vi "Config.vi"(8 "error in (no error)":errorcluster, 10 "Setting":variant, 11 "NI DMM in":refnum<class "NI DMM.lvclass">) -> (0 "error out":errorcluster, 3 "NI DMM out":refnum<class "NI DMM.lvclass">)   [LabVIEW 2025, in "DMM.lvlib" / "NI DMM.lvclass"]
uses:
  NI DMM.lvclass
  C:/Users/Public/Documents/Sandia National Labs/TSS Plugin/CEF.lvlibp/Node/CEF_Node.lvclass
  C:/Working copy/tss/Plugin/Engines/DMM/DMM Instrument/DMM Instrument.lvclass
  C:/Users/Public/Documents/Sandia National Labs/TSS Plugin/Abstract Engine.lvlibp/Abstract Instrument/Abstract Instrument.lvclass
  DMM configuration/DMM configuration.lvclass
  <instrlib>/niDMM/nidmm.llb/niDMM Function.ctl
  NI DMM.lvclass/NI DMM.ctl
  DMM configuration/DMM configuration.lvclass/DMM configuration.ctl
  <instrlib>/niDMM/nidmm.llb/niDMM Current Source.ctl
  <instrlib>/niDMM/nidmm.llb/niDMM Resolution in Digits.ctl
  Users/Public/Documents/Sandia National Labs/TSS Plugin/Abstract Engine.lvlibp/Abstract Instrument/Channel.ctl
  DMM Channel/DMM Channel.lvclass
  Users/Public/Documents/Sandia National Labs/TSS Plugin/Abstract Engine.lvlibp/Channel configuration/Channel configuration.lvclass
  DMM configuration/Read DMM Setting.vi
  Users/Public/Documents/Sandia National Labs/TSS Plugin/CEF.lvlibp/Node/ReadChildren.vi
  Users/Public/Documents/Sandia National Labs/TSS Plugin/Abstract Engine.lvlibp/Channel configuration/Read Channel Setting.vi
  <instrlib>/niDMM/nidmm.llb/niDMM Configure Measurement Digits.vi
  Users/Public/Documents/Sandia National Labs/TSS Plugin/CEF.lvlibp/Node/CEF_Node.lvclass
  Users/Public/Documents/Sandia National Labs/TSS Plugin/CEF.lvlibp/serializable configuration/CEF_serializable configuration.lvclass
  Users/Public/Documents/Sandia National Labs/TSS Plugin/Abstract Engine.lvlibp/Abstract Instrument/Abstract Instrument.lvclass
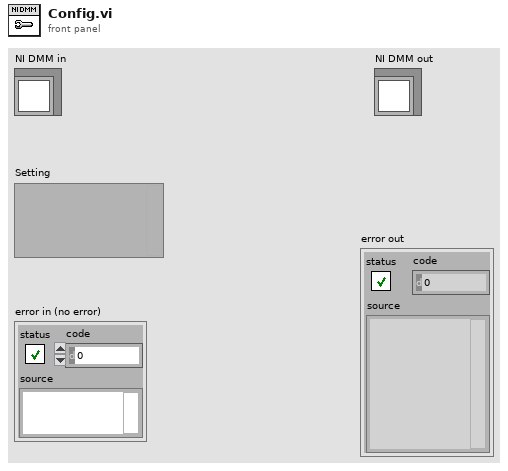
[diagram p1: front panel]
types:
  T1 = typedef "niDMM Function.ctl" = enum16{"DC Volts", "AC Volts", "DC Current", "AC Current", "2-wire Resistance", "4-wire Resistance", "Diode", "Frequency", "Period", "AC Volts DC Coupled", "Capacitance", "Inductance", "Temperature"}
  T2 = typedef "Abstract Engine.lvlibp/Abstract Instrument.lvclass/Channel.ctl" = cluster{"Alias":string, "DataType":enum16{"Anaolg Input", "Waveform"}, "Unit":enum16{"---", "V", "A", "Ohm", "Hz", "uF", "degC", "deg"}, "Upper limit":dbl, "Lower limit":dbl, "Measurement":variant}
  T3 = typedef "Abstract Engine.lvlibp/Channel configuration.lvclass/Default Channel.ctl" = cluster{"Address":string, "SW Alias":string, "Enabled":bool, "Type":string, "Description":string}
  T4 = typedef "DMM.lvlib/DMM configuration.lvclass/DMM Setting.ctl" = cluster{"Function":string, "CurrentSource":string, "Resolution":string, "Range":dbl}
  T5 = typedef "niDMM Resolution in Digits.ctl" = dbl
  T6 = typedef "niDMM Current Source.ctl" = dbl
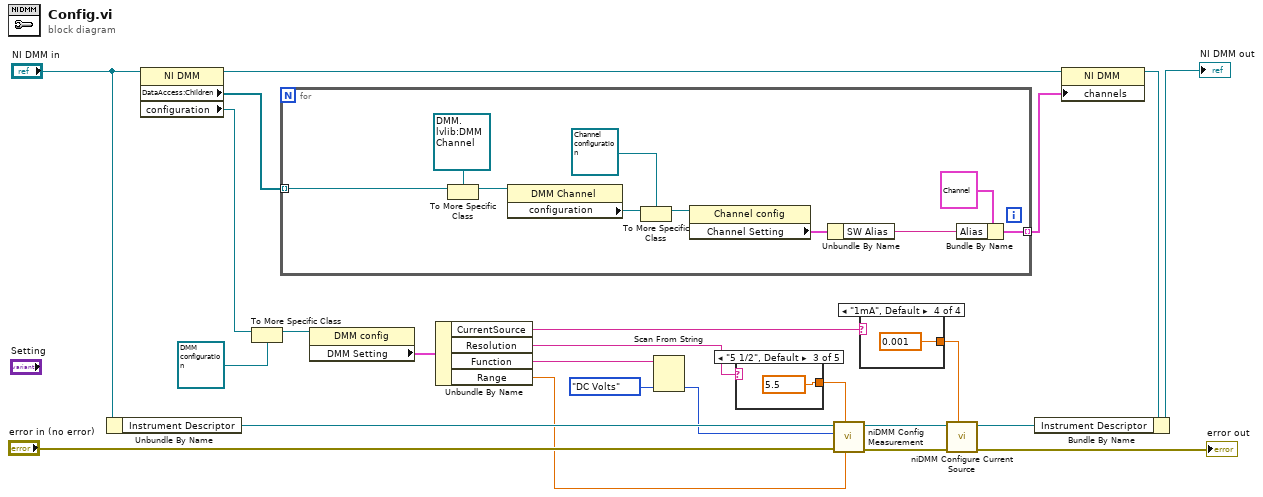
[diagram p0: block diagram]
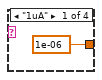
[diagram p2: hidden frame]
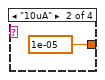
[diagram p3: hidden frame]
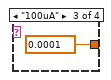
[diagram p4: hidden frame]
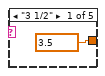
[diagram p5: hidden frame]
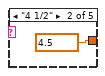
[diagram p6: hidden frame]
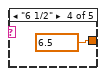
[diagram p7: hidden frame]
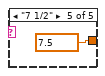
[diagram p8: hidden frame]
diagram:
  n1 = Unbundle By Name("NI DMM in") -> ("Instrument Descriptor"=w23:refnum<k15>)
  n2 = property class="NI DMM"(reference="NI DMM in") -> (reference out=w17:refnum<class "NI DMM.lvclass">, "DataAccess:Children"=w5:refnum<data-value>[], "configuration"=w6:refnum<class "CEF_serializable configuration.lvclass">)  [unwired: 1 in, 1 out]
  n3 = To More Specific Class(target class=refnum<class "DMM configuration.lvclass"> refnum ("DMM.lvlib:DMM configuration.lvclass"), reference=w6) -> (specific class reference=w19:refnum<class "DMM configuration.lvclass">)  [unwired: 1 in, 1 out]
  n4 = for {
    tunnel: w5 -> [w34] mode=indexing
    tunnel: [w32] -> w1 mode=indexing
    n5 = To More Specific Class(target class=refnum<data-value> refnum ("data value reference"), reference=w34) -> (specific class reference=w30:refnum<data-value>)  [unwired: 1 in, 1 out]
    n6 = property class="DMM Channel"(reference=w30) -> ("configuration"=w29:refnum<class "CEF_serializable configuration.lvclass">)  [unwired: 1 in, 2 out]
    n7 = To More Specific Class(target class=refnum<class "Channel configuration.lvclass"> refnum ("Abstract Engine.lvlibp:Channel config"), reference=w29) -> (specific class reference=w28:refnum<class "Channel configuration.lvclass">)  [unwired: 1 in, 1 out]
    n8 = property class="Channel config"(reference=w28) -> ("Channel Setting"=w27:T3)  [unwired: 1 in, 2 out]
    n9 = Unbundle By Name(w27) -> ("SW Alias"=w33:string)
    n10 = Bundle By Name(cluster=T2 {"Alias"="ch0", "DataType"=enum."Anaolg Input", "Unit"=enum."V", "Upper limit"=10.0, "Lower limit"=-10.0, "Measurement"=variant} ("Channel"), "Alias"=w33) -> (w32:T2)
  }
  n11 = property class="DMM config"(reference=w19) -> ("DMM Setting"=w8:T4)  [unwired: 1 in, 2 out]
  n12 = Unbundle By Name(w8) -> ("CurrentSource"=w9:string, "Resolution"=w11:string, "Function"=w4:string, "Range"=w2:dbl)
  n13 = Scan From String(input string=w4, default 1=niDMM_Function."DC Volts" ("Function")) -> (output 1=w3:T1)  [unwired: 3 in, 3 out]
  n14 = case shown="\"5 1/2\", Default" w11 {
    tunnel: [w35 w36 w37 w38 w39] -> w12
    frame "3 1/2" {
      w35 = T5 3.5 items=["3 1/2"=3.5, "4 1/2"=4.5, "5 1/2"=5.5, "6 1/2"=6.5, "7 1/2"=7.5] ("Resolution in Digits")
    }
    frame "4 1/2" {
      w36 = T5 4.5 items=["3 1/2"=3.5, "4 1/2"=4.5, "5 1/2"=5.5, "6 1/2"=6.5, "7 1/2"=7.5] ("Resolution in Digits")
    }
    frame "5 1/2", Default {
      w37 = T5 5.5 items=["3 1/2"=3.5, "4 1/2"=4.5, "5 1/2"=5.5, "6 1/2"=6.5, "7 1/2"=7.5] ("Resolution in Digits")
    }
    frame "6 1/2" {
      w38 = T5 6.5 items=["3 1/2"=3.5, "4 1/2"=4.5, "5 1/2"=5.5, "6 1/2"=6.5, "7 1/2"=7.5] ("Resolution in Digits")
    }
    frame "7 1/2" {
      w39 = T5 7.5 items=["3 1/2"=3.5, "4 1/2"=4.5, "5 1/2"=5.5, "6 1/2"=6.5, "7 1/2"=7.5] ("Resolution in Digits")
    }
  }
  n15 = call-poly <instrlib>:"niDMM Config Measurement.vi"("Range"=w2, "Resolution in Digits"=w12, "error in (no error)"="error in (no error)", "Function"=w3, "instrument handle"=w23) -> ("error out"=w14:errorcluster, "instrument handle out"=w20:refnum<k15>)  [unwired: 5 out]
  n16 = case shown="\"1mA\", Default" w9 {
    tunnel: [w40 w41 w42 w43] -> w10
    frame "1uA" {
      w40 = T6 1e-06 items=["1uA"=1e-06, "10uA"=1e-05, "100uA"=0.0001, "1mA"=0.001] ("Current Source")
    }
    frame "10uA" {
      w41 = T6 1e-05 items=["1uA"=1e-06, "10uA"=1e-05, "100uA"=0.0001, "1mA"=0.001] ("Current Source")
    }
    frame "100uA" {
      w42 = T6 0.0001 items=["1uA"=1e-06, "10uA"=1e-05, "100uA"=0.0001, "1mA"=0.001] ("Current Source")
    }
    frame "1mA", Default {
      w43 = T6 0.001 items=["1uA"=1e-06, "10uA"=1e-05, "100uA"=0.0001, "1mA"=0.001] ("Current Source")
    }
  }
  n17 = call <instrlib>:"niDMM Configure Current Source.vi"("Current Source"=w10, "error in (no error)"=w14, "instrument handle"=w20) -> ("error out"=→"error out":errorcluster, "instrument handle out"=w22:refnum<k15>)  [unwired: 1 in, 6 out]
  n18 = property class="NI DMM"(reference=w17, "channels"=w1) -> (reference out=w7:refnum<class "NI DMM.lvclass">)  [unwired: 1 in, 1 out]
  n19 = Bundle By Name(cluster=w7, "Instrument Descriptor"=w22) -> (→"NI DMM out":refnum<class "NI DMM.lvclass">)
